vi "AutoSaveTimer.vi"(3 "EN":bool, 4 "Time Delay (ms)":i32=1, 5 "Time Target (ms)":i32=1) -> (1 "Flash":bool)   [LabVIEW 2017]
panel:
  out "OLD":u32
  out "NEW":u32
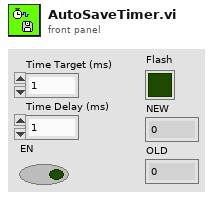
[diagram p1: front panel]
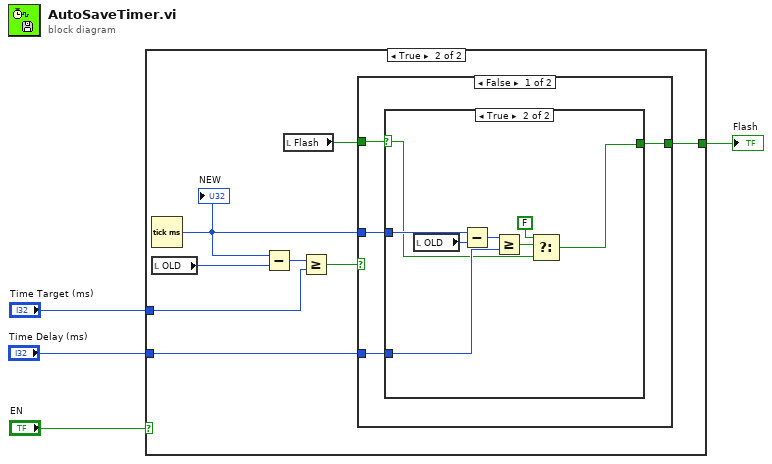
[diagram p0: block diagram]
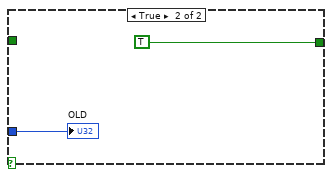
[diagram p4: hidden frame]
diagram:
  n1 = case shown="True" "EN" {
    tunnel: "Time Target (ms)" -> [_ w9]
    tunnel: [_ w7] -> w3
    tunnel: "Time Delay (ms)" -> [_ w5]
    frame False {
    }
    frame True {
      n2 = Tick Count (ms)() -> (millisecond timer value=w12:u32)
      "NEW" <- w12
      n3 = local read "OLD"() -> (w11:u32)
      n4 = Subtract(x=w12, y=w11) -> (x-y=w10:u32)
      n5 = local read "Flash"() -> (w6:bool)
      n6 = Greater Or Equal?(x=w10, y=w9) -> (x >= y?=w8:bool)
      n7 = case shown="False" w8 {
        tunnel: w12 -> [w14 w27]
        tunnel: [w15 TRUE ("Flash")] -> w7
        tunnel: w6 -> [w16 _]
        tunnel: w5 -> [w13 _]
        frame False {
          n8 = case shown="True" w16 {
            selector: w16 -> [w17 w20]
            tunnel: [w17 w19] -> w15
            tunnel: w14 -> [_ w25]
            tunnel: w13 -> [_ w22]
            frame False {
            }
            frame True {
              n9 = local read "OLD"() -> (w24:u32)
              n10 = Subtract(x=w25, y=w24) -> (x-y=w23:u32)
              n11 = Greater Or Equal?(x=w23, y=w22) -> (x >= y?=w21:bool)
              n12 = Select(t=FALSE, s=w21, f=w20) -> (s? t:f=w19:bool)
            }
          }
        }
        frame True {
          "OLD" <- w27
        }
      }
    }
  }
  "Flash" <- w3
